vi "Process Start Trial.vi"(11 "Matlab Param Array":cluster{"Name":string, "Data":variant}[](array[cluster])) -> (1 "allowSaccades":bool, 2 "acquireFixation":bool, 3 "passive":bool)   [LabVIEW 2009]
uses:
  Matlab API/Matlab Param Array to Boolean.vi
  Matlab API/Matlab API.lvlib
panel:
  out "error passive":errorcluster
  out "error fixation":errorcluster
  out "error saccades":errorcluster
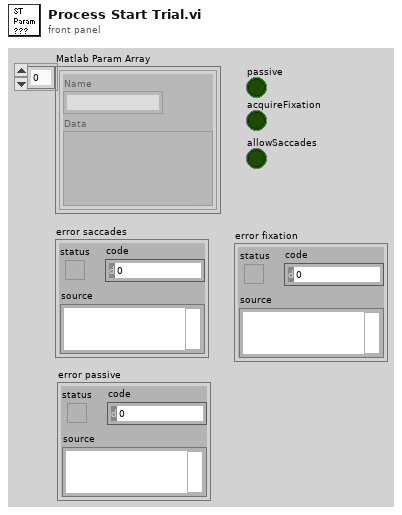
[diagram p1: front panel]
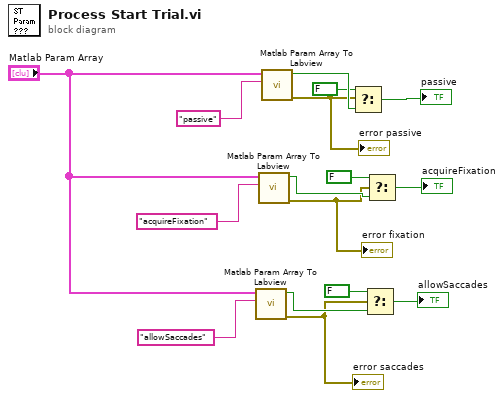
[diagram p0: block diagram]
diagram:
  n1 = call-poly "Matlab Param Array To Labview.vi"("Name"="allowSaccades", "Matlab Param Array"="Matlab Param Array") -> ("error out"=w7:errorcluster, "data"=w8:bool)  [unwired: 1 in, 7 out]
  "error saccades" <- w7
  n2 = call-poly "Matlab Param Array To Labview.vi"("Name"="acquireFixation", "Matlab Param Array"="Matlab Param Array") -> ("error out"=w2:errorcluster, "data"=w6:bool)  [unwired: 1 in, 7 out]
  "error fixation" <- w2
  n3 = call-poly "Matlab Param Array To Labview.vi"("Name"="passive", "Matlab Param Array"="Matlab Param Array") -> ("error out"=w1:errorcluster, "data"=w12:bool)  [unwired: 1 in, 7 out]
  "error passive" <- w1
  n4 = Select(t=FALSE, s=w1, f=w12) -> (s? t:f=→"passive":bool)
  n5 = Select(t=FALSE, s=w7, f=w8) -> (s? t:f=→"allowSaccades":bool)
  n6 = Select(t=FALSE, s=w2, f=w6) -> (s? t:f=→"acquireFixation":bool)
